vi "Setup NML Daq.vi"(7 "Input Limits":cluster{"High Limit":dbl, "Low Limit":dbl}[](array[cluster]) {"High Limit" format="%.3f"; "Low Limit" format="%.3g"}, 8 "rate":dbl=15000.0 format="%0.2f", 9 "number of samples per channel":i32=128, 10 "channels (0)":i32[](array[numeric])=[0, 1], 11 "Data Acq Device":string) -> (0 "error out":errorcluster, 3 "task out":refnum<k21>)   [LabVIEW 2021]
uses:
  <vilib>/_DAQmxBase/Internals/DAQmxBase Create Channel (AI-Voltage-Basic).vi
  <vilib>/_DAQmxBase/Internals/DAQmxBase Timing (Sample Clock).vi
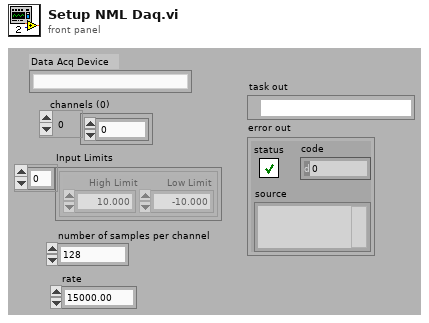
[diagram p1: front panel]
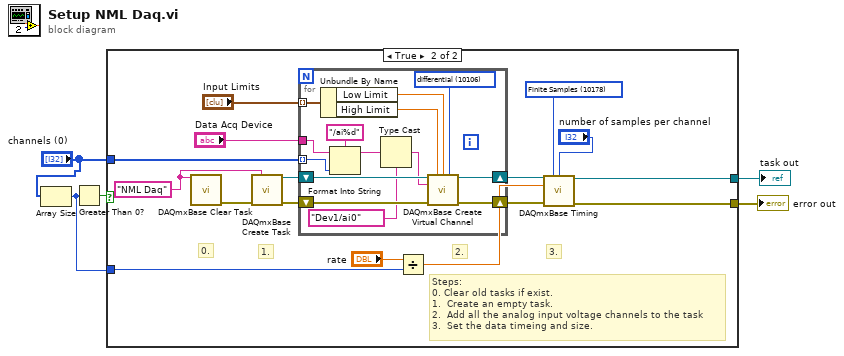
[diagram p0: block diagram]
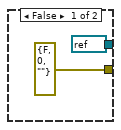
[diagram p2: hidden frame]
diagram:
  n1 = Array Size(array="channels (0)") -> (size(s)=w1:i32)
  n2 = Greater Than 0?(x=w1) -> (x > 0?=w2:bool)
  n3 = case shown="True" w2 {
    tunnel: [errorcluster {"status"=FALSE, "code"=0, "source"=""} ("error out") w16] -> w5
    tunnel: [refnum<k21> refnum ("task out") w15] -> w4
    tunnel: "channels (0)" -> [_ w14]
    tunnel: w1 -> [_ w8]
    frame False {
    }
    frame True {
      w13 = "NML Daq" ("new task name")
      w18 = 10178 items=["Finite Samples"=10178, "Continuous Samples"=10123, "Hardware Timed Single Point"=12522] ("sample mode")
      # "0."
      # "3."
      # "2."
      # "1."
      # "Steps: \n0. Clear old tasks if exist.\n1.  Create an empty task.\n2.  Add all the analog input voltage channels to the task\n3.  Set the data timeing and size."
      n4 = call <vilib>:"DAQmxBase Clear Task.vi"("task in"=w13) -> ("error out"=w12:errorcluster)  [unwired: 14 in]
      n5 = call <vilib>:"DAQmxBase Create Task.vi"("new task name"=w13, "error in"=w12) -> ("task out"=w23:refnum<k21>, "error out"=w22:errorcluster)  [unwired: 12 in]
      n6 = for {
        tunnel: "Input Limits" -> [w37] mode=indexing
        tunnel: w14 -> [w29] mode=indexing
        shift-right: [w34] -> w21
        shift-left: w23 -> [w36]
        shift-right: [w33] -> w20
        shift-left: w22 -> [w35]
        tunnel: "Data Acq Device" -> [w28]
        w24 = 10106 items=["default"=-1, "differential"=10106, "RSE"=10083, "NRSE"=10078] ("input terminal configuration")
        n7 = Unbundle By Name(w37) -> ("Low Limit"=w32:dbl, "High Limit"=w31:dbl)
        n8 = Format Into String(format string="/ai%d", initial string=w28, w29) -> (resulting string=w30:string)  [unwired: 1 in, 1 out]
        n9 = Type Cast(type=tag "Dev1/ai0" ("Physical Channel 2"), x=w30) -> (*(type *) &x=w26:tag)
        n10 = call-poly <vilib>:"DAQmxBase Create Virtual Channel.vi"("task in"=w36, "maximum value"=w31, "minimum value"=w32, "input terminal configuration"=w24, "physical channels"=w26, "error in"=w35) -> ("task out"=w34:refnum<k21>, "error out"=w33:errorcluster)  [unwired: 8 in]
      }
      n11 = Divide(x="rate", y=w8) -> (x/y=w9:dbl)
      n12 = call-poly <vilib>:"DAQmxBase Timing.vi"("task/channels in"=w21, "sample mode"=w18, "samples per channel"="number of samples per channel", "rate"=w9, "error in"=w20) -> ("task out"=w15:refnum<k21>, "error out"=w16:errorcluster)  [unwired: 9 in]
    }
  }
  "task out" <- w4
  "error out" <- w5
